vi "Test Work Dispatcher Forward Message When Adding Worker.vi"(8 "error in (no error)":errorcluster, 11 "Work Dispatcher Test in":refnum<class "Work Dispatcher Test.lvclass">) -> (0 "error out":errorcluster, 3 "Work Dispatcher Test out":refnum<class "Work Dispatcher Test.lvclass">)   [LabVIEW 2020, in "Work Dispatcher Test.lvclass"]
uses:
  Work Dispatcher Test.lvclass
  C:/Program Files (x86)/National Instruments/LabVIEW 2020/vi.lib/Asteme/LUnit/Test Case.lvclass
  Work Dispatcher/Work Dispatcher.lvclass
  C:/Program Files (x86)/National Instruments/LabVIEW 2020/vi.lib/Asteme/Triarc Framework/Process/Process.lvclass
  Mock Worker/Mock Worker.lvclass
  C:/Users/anton/Documents/GitHub/Triarc-Examples/Coffee Shop/Process Job/Process Job.lvclass
  <vilib>/Asteme/Triarc Framework/Process/Process.lvclass
  <vilib>/Asteme/Triarc Framework/Process/Process.lvclass/Process.ctl
  <vilib>/Asteme/LUnit/Test Case.lvclass/Test Case.ctl
  <vilib>/Asteme/LUnit/LUnit Assertion Result.lvclass/LUnit Assertion Result.ctl
  <vilib>/Asteme/Triarc Framework Test Suite/Support/Execution timer.vi
  <vilib>/Asteme/Triarc Framework/Process/Private/SubVIs/Wait for finish.vi
  <vilib>/Asteme/Triarc Framework/Process/Protected/Messaging/Enqueue Message.vi
  <vilib>/Asteme/Triarc Framework/Process/Private/SubVIs/Set Lifecycle State.vi
  <vilib>/Asteme/Triarc Framework/Process/Public/Lifecycle/Get Lifecycle State.vi
  <vilib>/Asteme/LUnit/Palette/Fail.vi
  <vilib>/Asteme/LUnit/Palette/Pass.vi
  <vilib>/Asteme/LUnit/Set Assertion Type.vi
  <vilib>/Utility/error.llb/Clear Errors.vi
  <vilib>/Asteme/LUnit/Add test result.vi
  <vilib>/Asteme/LUnit/LUnit Write Passed.vi
  <vilib>/Asteme/LUnit/LUnit Get Test Case.vi
  <vilib>/Asteme/LUnit/Assertion Result/LUnit Get Test Name.vi
  <vilib>/Asteme/LUnit/LUnit Write Message.vi
  <vilib>/Asteme/LUnit/LUnit Write Description.vi
  <vilib>/Asteme/LUnit/LUnit Write Assertion Type.vi
  <vilib>/Asteme/LUnit/Read Test Case Name.vi
  <vilib>/Asteme/Triarc Framework Test Suite/Support/Event Helpers/Dequeue Event Message.vi
  <vilib>/Utility/error.llb/Error Cluster From Error Code.vi
  <vilib>/Asteme/LUnit/LUnit Assertion Result.lvclass
  C:/Program Files (x86)/National Instruments/LabVIEW 2020/vi.lib/Asteme/Triarc Framework/Base/Base.lvclass
  C:/Program Files (x86)/National Instruments/LabVIEW 2020/vi.lib/Asteme/Triarc Framework/Error Handler Interface/Error Handler Interface.lvclass
  C:/Program Files (x86)/National Instruments/LabVIEW 2020/vi.lib/Asteme/Triarc Framework/Logging/Logging.lvclass
  C:/Users/anton/Documents/GitHub/Triarc-Examples/Coffee Shop/Work Dispatcher/Work Dispatcher.lvclass
  C:/Program Files (x86)/National Instruments/LabVIEW 2020/vi.lib/Asteme/Triarc Framework/Helper Loop/Helper Loop.lvclass
  <vilib>/Asteme/Triarc Framework Test Suite/Support/Event Helpers/Event Helpers.lvlib
  <vilib>/Asteme/LUnit/Test Case.lvclass
  C:/Program Files (x86)/National Instruments/LabVIEW 2020/vi.lib/Asteme/Triarc Framework Test Suite/Process Test/Process Test.lvclass
  C:/Program Files (x86)/National Instruments/LabVIEW 2020/vi.lib/Asteme/Triarc Framework Test Suite/Base Class Test/Base Test.lvclass
  C:/Users/anton/Documents/GitHub/Triarc-Examples/Coffee Shop/Work Dispatcher Test/Work Dispatcher Test.lvclass
  C:/Users/anton/Documents/GitHub/Triarc-Examples/Coffee Shop/Mock Worker/Mock Worker.lvclass
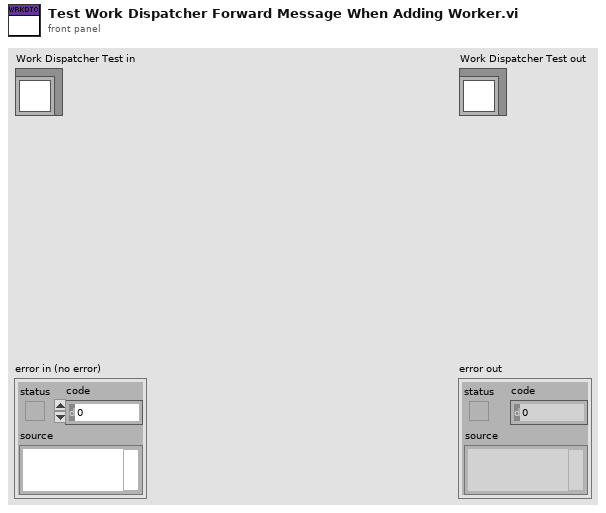
[diagram p1: front panel]
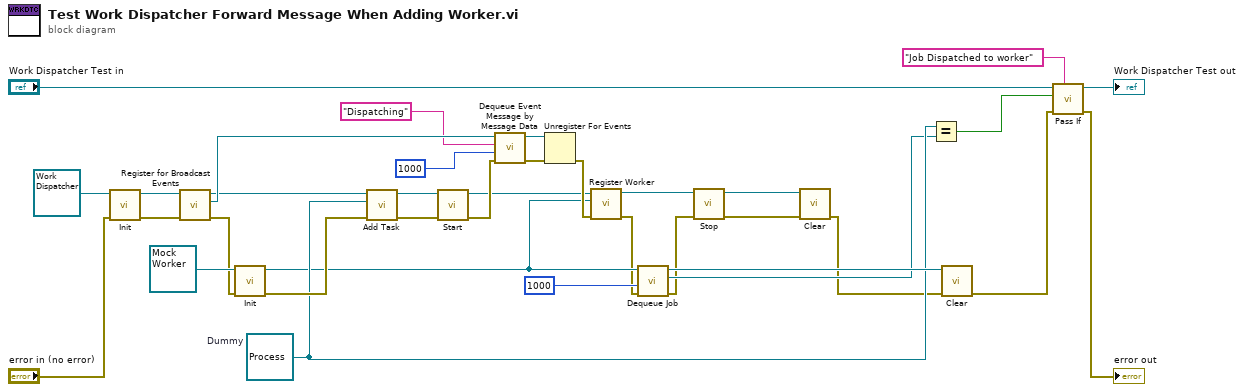
[diagram p0: block diagram]
diagram:
  w14 = refnum<class "Process.lvclass"> refnum  # Dummy
  n1 = call-dynamic "Init.vi"("error in (no error)"="error in (no error)", "Process In"=refnum<class "Work Dispatcher.lvclass"> refnum ("Work Dispatcher.lvclass")) -> ("error out"=w32:errorcluster, "Process Out"=w33:refnum<class "Work Dispatcher.lvclass">)  [unwired: 8 in]
  n2 = call <vilib>:"Register for Broadcast Events.vi"("error in (no error)"=w32, "Process In"=w33) -> ("error out"=w19:errorcluster, "Event Registration Refnum Out"=w27:refnum<event-registration>, "Process Out"=w20:refnum<class "Work Dispatcher.lvclass">)  [unwired: 7 in]
  n3 = call-dynamic "Init.vi"("error in (no error)"=w19, "Mock Worker In"=refnum<class "Mock Worker.lvclass"> refnum) -> ("error out"=w18:errorcluster, "Mock Worker Out"=w5:refnum<class "Mock Worker.lvclass">)  [unwired: 8 in]
  n4 = call "Add Task.vi"("error in (no error)"=w18, "Task"=w14, "Work Dispatcher In"=w20) -> ("error out"=w16:errorcluster, "Work Dispatcher Out"=w17:refnum<class "Work Dispatcher.lvclass">)  [unwired: 7 in]
  n5 = call <vilib>:"Start.vi"("error in (no error)"=w16, "Process In"=w17) -> ("error out"=w24:errorcluster, "Process Out"=w7:refnum<class "Work Dispatcher.lvclass">)  [unwired: 8 in]
  n6 = call <vilib>:"Dequeue Event Message by Message Data.vi"("error in (no error)"=w24, "Timeout (-1)"=1000, "Message Data"="Dispatching", "Event Registration Refnum"=w27) -> ("error out"=w23:errorcluster, "Event Registration Refnum Out"=w21:refnum<event-registration>)  [unwired: 3 in, 3 out]
  n7 = Unregister For Events(event registration refnum=w21, error in=w23) -> (error out=w22:errorcluster)
  n8 = call "Register Worker.vi"("error in (no error)"=w22, "Worker"=w5, "Work Dispatcher In"=w7) -> ("error out"=w3:errorcluster, "Work Dispatcher Out"=w6:refnum<class "Work Dispatcher.lvclass">)  [unwired: 7 in]
  n9 = call "Dequeue Job.vi"("error in (no error)"=w3, "timeout in ms (-1)"=1000, "Mock Worker in"=w5) -> ("error out"=w2:errorcluster, "element"=w13:refnum<class>, "Mock Worker out"=w28:refnum<class "Mock Worker.lvclass">)  [unwired: 5 in, 1 out]
  n10 = call <vilib>:"Stop.vi"("error in (no error)"=w2, "Process In"=w6) -> ("error out"=w30:errorcluster, "Process Out"=w31:refnum<class "Work Dispatcher.lvclass">)  [unwired: 7 in, 1 out]
  n11 = call-dynamic "Clear.vi"("error in (no error)"=w30, "Process In"=w31) -> ("error out"=w1:errorcluster)  [unwired: 9 in]
  n12 = Equal?(x=w14, y=w13) -> (x = y?=w10:bool)
  n13 = call-dynamic "Clear.vi"("error in (no error)"=w1, "Mock Worker In"=w28) -> ("error out"=w9:errorcluster)  [unwired: 9 in]
  n14 = call <vilib>:"Pass If.vi"("Description"="Job Dispatched to worker", "error in (no error)"=w9, "Pass?"=w10, "Test Case In"="Work Dispatcher Test in") -> ("error out"=→"error out":errorcluster, "Test Case Out"=→"Work Dispatcher Test out":refnum<class "Work Dispatcher Test.lvclass">)  [unwired: 6 in]
